vi "CSM - Destroy Status Change Event.vi"(8 "Error In":errorcluster caption="error in (no error)", 11 "Status Change Event":refnum<user-event>) -> (0 "error out":errorcluster)   [LabVIEW 2017, in "Communicable State Machine.lvlib"]
doc: "### CSM - Destroy Status Change Event.vi\n\nRelease the CSM status change event handle.\n\n-- <b>Controls</b> --\n- <b>Status Change Event</b>: CSM status change event handle"
uses:
  _Support/Typedef/_CSM Status Change Event Data.ctl
  Communicable State Machine.lvlib
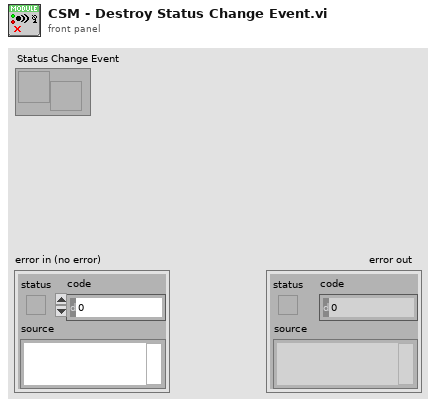
[diagram p1: front panel]
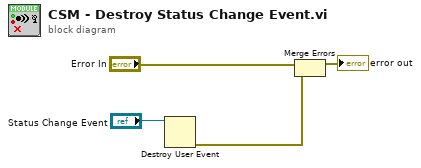
[diagram p0: block diagram]
diagram:
  n1 = Destroy User Event(user event="Status Change Event") -> (error out=w4:errorcluster)  [unwired: 1 in]
  n2 = Merge Errors("Error In", w4) -> (→"error out":errorcluster)
